vi "Express VI String Globals.vi"() -> ()   [LabVIEW 2021]
panel:
  in  "AO.NodeDescription":string="This Express VI writes values to the selected channels."
  in  "AO.NodeTitle":string="AO Write"
  in  "AI.NodeDescription":string="This Express VI reads values of selected channels."
  in  "AI.NodeTitle":string="AI Read"
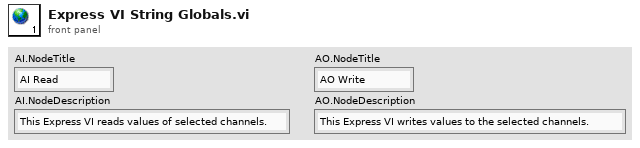
[diagram p1: front panel]
diagram:
